vi "Formula.vi"   [LabVIEW 2014]
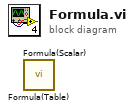
[diagram p0: block diagram]
diagram:
  n1 = call "Formula(Table).vi"() -> ()  [unwired: 10 in, 2 out]
  n2 = call "Formula(Scalar).vi"() -> ()  [unwired: 10 in, 2 out]
